vi "DiffIO Read.vi"(7 "Device Outputs in":dbl[](array[numeric]), 8 "FIFO Indexes.Read":T3, 9 "Command Enabled":bool, 10 "Diff IO Results":T4[](array[typedef]) {"Duty Cycle [%]" format="%#_3g"; "Frequency [Hz]" format="%#_3p"}, 11 "Diff I/O In":T1) -> (5 "Device Outputs out":dbl[](array[numeric]))   [LabVIEW 2016, in "DCM Engine.lvlib"]
uses:
  DCM Engine.lvlib
  Built/DCM Classes Packed/Pharlap/C/DCM-Classes.lvlibp/DCM/Diff IO/RT/Results.ctl
  Shared/Types/DiffIO Results Indexes.ctl
  <vilib>/Powertrain Controls/Device Drivers/DCM/Tools/FPGA/8 Channels.ctl
  DCM Shared.lvlib
  Built/DCM Classes Packed/Pharlap/C/DCM-Classes.lvlibp/DCM/Diff IO/RT/DCM - RT - Diff IO.lvlib
  <vilib>/Powertrain Controls/Device Drivers/DCM/Tools/FPGA/DCM - FPGA - Tools.lvlib
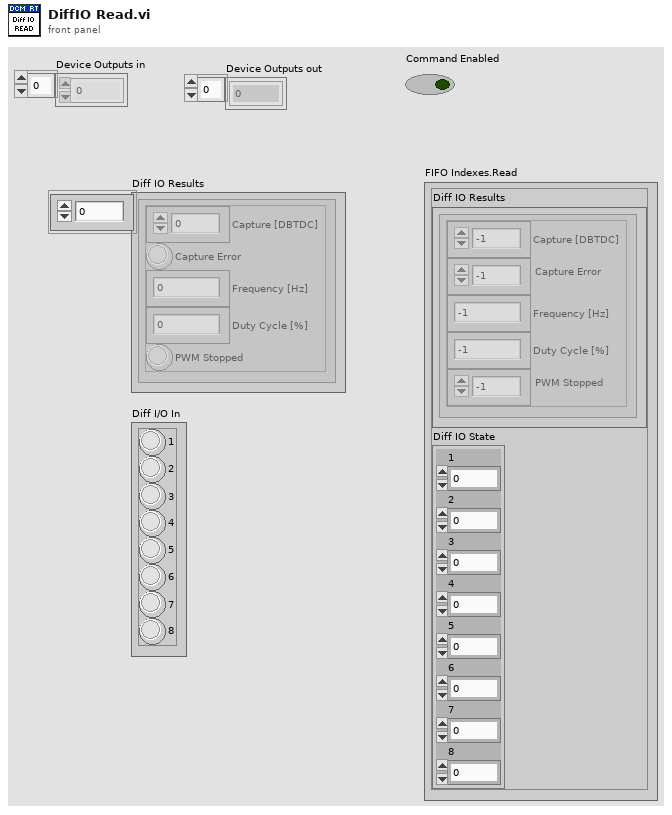
[diagram p1: front panel]
types:
  T1 = typedef "DCM - FPGA - Tools.lvlib/8 Channels.ctl" = cluster{"1":bool, "2":bool, "3":bool, "4":bool, "5":bool, "6":bool, "7":bool, "8":bool}
  T2 = typedef "DCM Shared.lvlib/DiffIO Results Indexes.ctl" = cluster{"Capture [DBTDC]":i32, "Capture Error":i32, "Frequency [Hz]":i32, "Duty Cycle [%]":i32, "PWM Stopped":i32}
  T3 = cluster{"Diff IO Results":T2[], "Diff IO State":cluster{"1":i32, "2":i32, "3":i32, "4":i32, "5":i32, "6":i32, "7":i32, "8":i32}}
  T4 = typedef "DCM-Classes.lvlibp/DCM - RT - Diff IO.lvlib/Results.ctl" = cluster{"Capture [DBTDC]":sgl, "Capture Error":bool, "Frequency [Hz]":sgl, "Duty Cycle [%]":sgl, "PWM Stopped":bool}
  T5 = cluster{"1":i32, "2":i32, "3":i32, "4":i32, "5":i32, "6":i32, "7":i32, "8":i32}
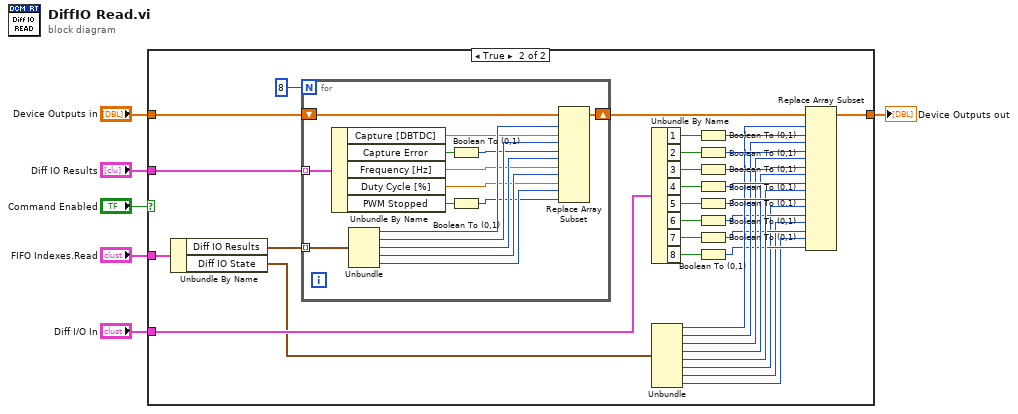
[diagram p0: block diagram]
diagram:
  n1 = case shown="True" "Command Enabled" {
    tunnel: [w7 w10] -> w6
    tunnel: "Device Outputs in" -> [w7 w40]
    tunnel: "FIFO Indexes.Read" -> [_ w39]
    tunnel: "Diff IO Results" -> [_ w38]
    tunnel: "Diff I/O In" -> [_ w9]
    frame False {
    }
    frame True {
      n2 = Unbundle By Name(w39) -> ("Diff IO Results"=w37:T2[], "Diff IO State"=w8:T5)
      n3 = for {
        N: 8 -> [_]
        tunnel: w38 -> [w47] mode=indexing
        tunnel: w37 -> [w46] mode=indexing
        shift-right: [w44] -> w11
        shift-left: w40 -> [w45]
        n4 = Unbundle By Name(w47) -> ("Capture [DBTDC]"=w41:sgl, "Capture Error"=w48:bool, "Frequency [Hz]"=w42:sgl, "Duty Cycle [%]"=w43:sgl, "PWM Stopped"=w49:bool)
        n5 = Unbundle(w46) -> ("Capture [DBTDC]"=w52:i32, "Capture Error"=w53:i32, "Frequency [Hz]"=w54:i32, "Duty Cycle [%]"=w55:i32, "PWM Stopped"=w56:i32)
        n6 = Boolean To (0,1)(Boolean=w48) -> (0, 1=w50:i16)
        n7 = Boolean To (0,1)(Boolean=w49) -> (0, 1=w51:i16)
        n8 = Replace Array Subset(array=w45, new element #1=w41, index #1=w52, new element #2=w50, index #2=w53, new element #3=w42, index #3=w54, new element #4=w43, index #4=w55, new element #5=w51, index #5=w56) -> (w44:dbl[])
      }
      n9 = Unbundle By Name(w9) -> ("1"=w31:bool, "2"=w35:bool, "3"=w34:bool, "4"=w33:bool, "5"=w32:bool, "6"=w20:bool, "7"=w19:bool, "8"=w18:bool)
      n10 = Unbundle(w8) -> ("1"=w25:i32, "2"=w24:i32, "3"=w23:i32, "4"=w22:i32, "5"=w21:i32, "6"=w14:i32, "7"=w13:i32, "8"=w12:i32)
      n11 = Boolean To (0,1)(Boolean=w31) -> (0, 1=w30:i16)
      n12 = Boolean To (0,1)(Boolean=w35) -> (0, 1=w29:i16)
      n13 = Boolean To (0,1)(Boolean=w34) -> (0, 1=w28:i16)
      n14 = Boolean To (0,1)(Boolean=w33) -> (0, 1=w26:i16)
      n15 = Boolean To (0,1)(Boolean=w32) -> (0, 1=w27:i16)
      n16 = Boolean To (0,1)(Boolean=w20) -> (0, 1=w17:i16)
      n17 = Boolean To (0,1)(Boolean=w19) -> (0, 1=w16:i16)
      n18 = Boolean To (0,1)(Boolean=w18) -> (0, 1=w15:i16)
      n19 = Replace Array Subset(array=w11, new element #1=w30, index #1=w25, new element #2=w29, index #2=w24, new element #3=w28, index #3=w23, new element #4=w26, index #4=w22, new element #5=w27, index #5=w21, new element #6=w17, index #6=w14, new element #7=w16, index #7=w13, new element #8=w15, index #8=w12) -> (w10:dbl[])
    }
  }
  "Device Outputs out" <- w6
